vi "AMZ_S3_APIHLP_Parse Setup RequestPayent Parameters.vi"(8 "error in (no error)":errorcluster, 11 "RequestPaymentConfiguration":T1) -> (0 "error out":errorcluster, 5 "PUT Data":string)   [LabVIEW 2015, in "LV Interface for Amazon S3.lvlib"]
uses:
  LV Interface for Amazon S3.lvlib
  Typedefs/AMZ_S3_API_RequestPaymentConfig.ctl
  Typedefs/AMZ_S3_Payer.ctl
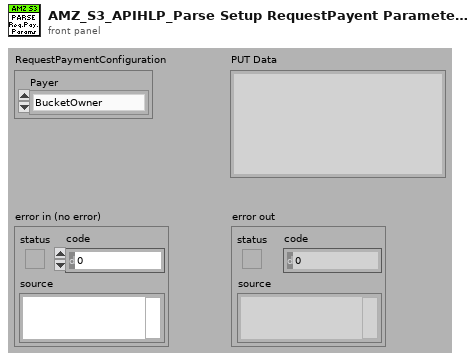
[diagram p1: front panel]
types:
  T1 = typedef "LV Interface for Amazon S3.lvlib/AMZ_S3_API_RequestPaymentConfig.ctl" = cluster{"Payer":T2}
  T2 = typedef "LV Interface for Amazon S3.lvlib/AMZ_S3_Payer.ctl" = enum16{"BucketOwner", "Requester"}
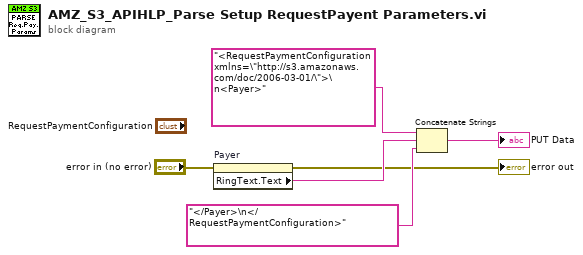
[diagram p0: block diagram]
diagram:
  n1 = property on="Payer" class="Enum (strict)"(error in="error in (no error)") -> (error out=→"error out":errorcluster, "RingText.Text"=w4:string)  [unwired: 1 in, 1 out]
  n2 = Concatenate Strings("<RequestPaymentConfiguration xmlns=\"http://s3.amazonaws.com/doc/2006-03-01/\">\n<Payer>", w4, "</Payer>\n</RequestPaymentConfiguration>") -> (→"PUT Data":string)
